vi "Read Experiment Description.vi"(8 "error in (no error)":errorcluster, 11 "Control Experiment in":refnum<class "Control Experiment SM.lvclass">) -> (0 "error out":errorcluster, 2 "Experiment Description":string, 3 "Control Experiment out":refnum<class "Control Experiment SM.lvclass">)   [LabVIEW 2016, in "Control Experiment SM.lvclass"]
uses:
  Control Experiment SM/Control Experiment SM.lvclass
  Control Experiment SM/Control Experiment SM.lvclass/Control Experiment SM.ctl
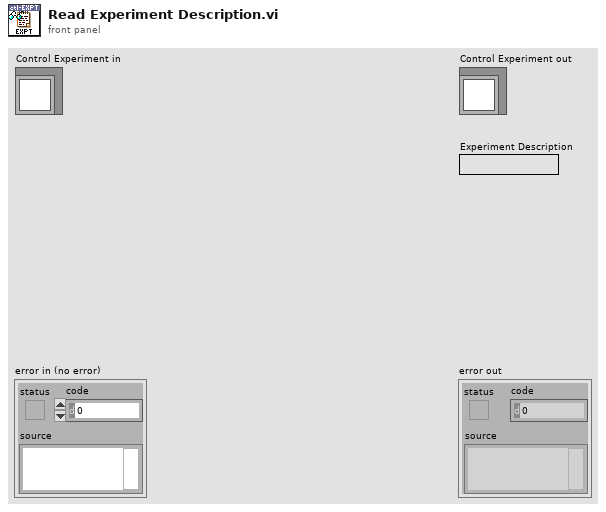
[diagram p1: front panel]
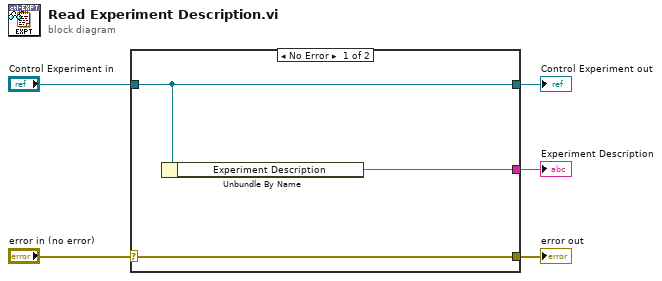
[diagram p0: block diagram]
diagram:
  n1 = case shown="No Error" "error in (no error)" {
    selector: "error in (no error)" -> [w8 w9]
    tunnel: [w8 w9] -> w4
    tunnel: [w7 w10] -> w2
    tunnel: "Control Experiment in" -> [w7 w10]
    tunnel: [w6 _] -> w1
    frame No Error {
      n2 = Unbundle By Name(w7) -> ("Experiment Description"=w6:string)
    }
    frame Error {
    }
  }
  "error out" <- w4
  "Control Experiment out" <- w2
  "Experiment Description" <- w1
